vi "Generate Sine Tone.vi"(0 "tone frequency":dbl format="%#_13p", 5 "amplitude":dbl=0.9 format="%#_13g", 7 "sample rate":dbl=3072000000.0 format="%#_13p") -> (4 "data out":cdb[](array[numeric]))   [LabVIEW 2019]
uses:
  <vilib>/Analysis/NI_AALBase.lvlib
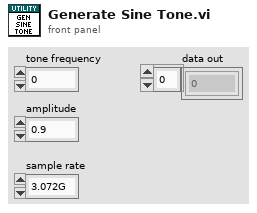
[diagram p1: front panel]
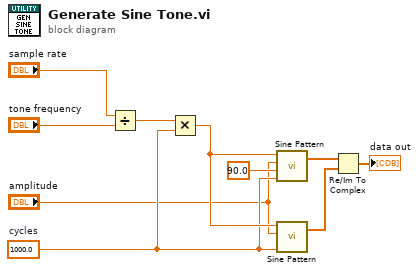
[diagram p0: block diagram]
diagram:
  w9 = 1000.0  # cycles
  n1 = Divide(x="sample rate", y="tone frequency") -> (x/y=w8:dbl)
  n2 = Multiply(x=w8, y=w9) -> (x*y=w10:dbl)
  n3 = call <vilib>:"Sine Pattern.vi"("cycles"=w9, "phase(degrees)"=90.0, "amplitude"="amplitude", "samples"=w10) -> ("Sinusoidal Pattern"=w3:dbl[])  [unwired: 1 out]
  n4 = call <vilib>:"Sine Pattern.vi"("cycles"=w9, "amplitude"="amplitude", "samples"=w10) -> ("Sinusoidal Pattern"=w4:dbl[])  [unwired: 1 in, 1 out]
  n5 = Re/Im To Complex(1:w4, 2:w3) -> (0:→"data out":cdb[])
